vi "Frame Set Basic Data.vi"(8 "error in (no error)":errorcluster, 10 "Frame Basic Data":T1, 11 "IDE simple in":refnum<class "Main Panel.lvclass">) -> (0 "error out":errorcluster, 3 "IDE simple out":refnum<class "Main Panel.lvclass">)   [LabVIEW 2018, in "Main Panel.lvlib" / "Main Panel.lvclass"]
uses:
  Main Panel.lvclass
  Frame Analizer/frame basic data.ctl
  Main Panel.lvclass/Main Panel.ctl
  Frame Analizer/Data Parser.lvclass
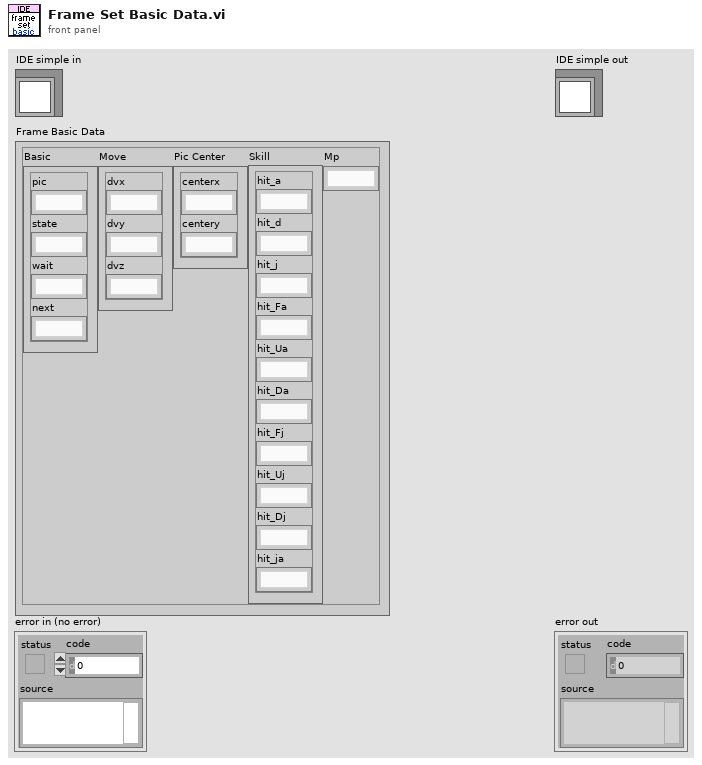
[diagram p1: front panel]
types:
  T1 = typedef "Data Parser.lvclass/frame basic data.ctl" = cluster{"Basic":cluster{"pic":string, "state":string, "wait":string, "next":string}, "Move":cluster{"dvx":string, "dvy":string, "dvz":string}, "Pic Center":cluster{"centerx":string, "centery":string}, "Skill":cluster{"hit_a":string, "hit_d":string, "hit_j":string, "hit_Fa":string, "hit_Ua":string, "hit_Da":string, "hit_Fj":string, "hit_Uj":string, "hit_Dj":string, "hit_ja":string}, "Mp":string}
  T2 = cluster{"centerx":refnum<vi>, "centery":refnum<vi>}
  T3 = cluster{"dvx":refnum<vi>, "dvy":refnum<vi>, "dvz":refnum<vi>}
  T4 = cluster{"hit_a":refnum<vi>, "hit_d":refnum<vi>, "hit_j":refnum<vi>, "hit_Fa":refnum<vi>, "hit_Ua":refnum<vi>, "hit_Da":refnum<vi>, "hit_Fj":refnum<vi>, "hit_Uj":refnum<vi>, "hit_Dj":refnum<vi>, "hit_ja":refnum<vi>}
  T5 = cluster{"dvx":string, "dvy":string, "dvz":string}
  T6 = cluster{"hit_a":string, "hit_d":string, "hit_j":string, "hit_Fa":string, "hit_Ua":string, "hit_Da":string, "hit_Fj":string, "hit_Uj":string, "hit_Dj":string, "hit_ja":string}
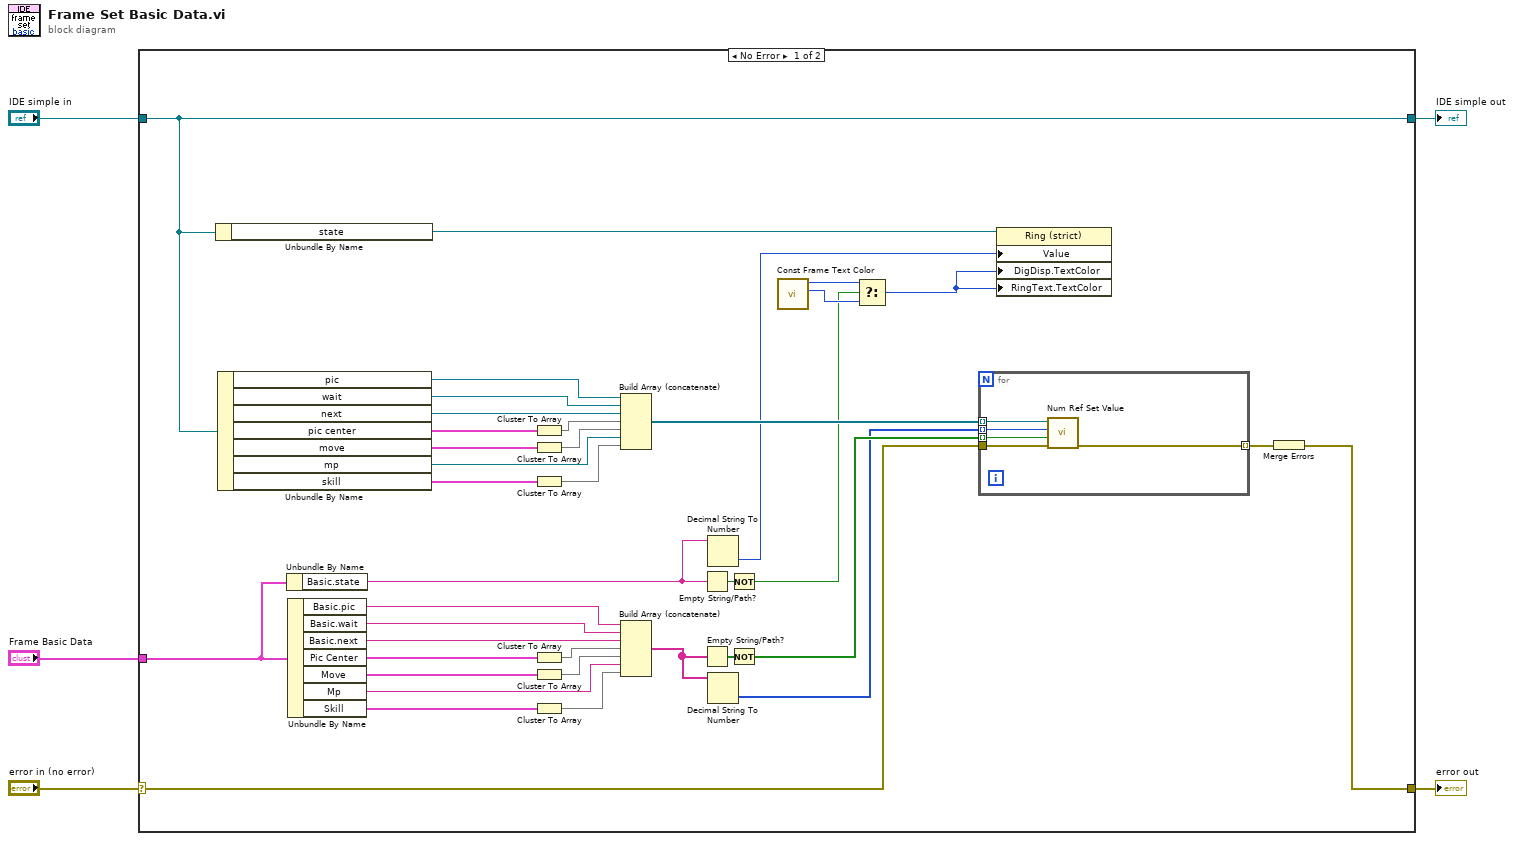
[diagram p0: block diagram]
diagram:
  n1 = case shown="No Error" "error in (no error)" {
    selector: "error in (no error)" -> [w42 w50]
    tunnel: [w22 w50] -> w4
    tunnel: [w21 w49] -> w2
    tunnel: "IDE simple in" -> [w21 w49]
    tunnel: "Frame Basic Data" -> [w10 _]
    frame No Error {
      n2 = Unbundle By Name(w21) -> ("state"=w17:refnum<vi>)
      n3 = Unbundle By Name(w21) -> ("pic"=w20:refnum<vi>, "wait"=w19:refnum<vi>, "next"=w18:refnum<vi>, "pic center"=w41:T2, "move"=w40:T3, "mp"=w36:refnum<vi>, "skill"=w39:T4)
      n4 = Unbundle By Name(w10) -> ("Basic.state"=w8:string)
      n5 = Unbundle By Name(w10) -> ("Basic.pic"=w13:string, "Basic.wait"=w12:string, "Basic.next"=w11:string, "Pic Center"=w34:cluster{"centerx":string, "centery":string}, "Move"=w33:T5, "Mp"=w29:string, "Skill"=w32:T6)
      n6 = Cluster To Array(cluster=w41) -> (array=w38:refnum<vi>[])
      n7 = Cluster To Array(cluster=w40) -> (array=w37:refnum<vi>[])
      n8 = Cluster To Array(cluster=w39) -> (array=w35:refnum<vi>[])
      n9 = Cluster To Array(cluster=w34) -> (array=w31:string[])
      n10 = Cluster To Array(cluster=w33) -> (array=w30:string[])
      n11 = Cluster To Array(cluster=w32) -> (array=w28:string[])
      n12 = Build Array (concatenate)(w20, w19, w18, w38, w37, w36, w35) -> (w26:refnum<vi>[])
      n13 = Build Array (concatenate)(w13, w12, w11, w31, w30, w29, w28) -> (w27:string[])
      n14 = Empty String/Path?(string/path=w8) -> (empty?=w9:bool)
      n15 = Empty String/Path?(string/path=w27) -> (empty?=w43:bool[])
      n16 = Decimal String To Number(string=w8) -> (number=w6:i32)  [unwired: 2 in, 1 out]
      n17 = Decimal String To Number(string=w27) -> (number=w24:i32[])  [unwired: 2 in, 1 out]
      n18 = Not(x=w9) -> (.not. x?=w7:bool)
      n19 = Not(x=w43) -> (.not. x?=w25:bool[])
      n20 = call "Const Frame Text Color.vi"() -> ("invalid num color"=w15:u32, "valid num color"=w16:u32)  [unwired: 10 in]
      n21 = Select(t=w16, s=w7, f=w15) -> (s? t:f=w14:u32)
      n22 = for {
        tunnel: w42 -> [w48]
        tunnel: w26 -> [w44] mode=indexing
        tunnel: w25 -> [w47] mode=indexing
        tunnel: w24 -> [w46] mode=indexing
        tunnel: [w45] -> w23 mode=indexing
        n23 = call "Num Ref Set Value.vi"("error in"=w48, "Valid"=w47, "Value"=w46, "Num Ref"=w44) -> ("error out"=w45:errorcluster)  [unwired: 7 in]
      }
      n24 = property class="Ring (strict)"(reference=w17, "Value"=w6, "DigDisp.TextColor"=w14, "RingText.TextColor"=w14) -> ()  [unwired: 1 in, 2 out]
      n25 = Merge Errors(w23) -> (w22:errorcluster)
    }
    frame Error {
    }
  }
  "error out" <- w4
  "IDE simple out" <- w2
